vi "sub_list_all_devices_for_user_flat_output.vi"(8 "error in (no error)":errorcluster, 11 "daq.io type in":T2={"daq.io ref"=refnum, "daq.io API Base"="http://dashboard.daq.io/api/v1", "Device Type Key"="", "Device Key"="", "Account ID"="", "online"=FALSE, "SSL"=TRUE}) -> (0 "error out":errorcluster, 2 "List of Devices":T1[](array[typedef]), 3 "daq.io type out":T2={"daq.io ref"=refnum, "daq.io API Base"="http://dashboard.daq.io/api/v1", "Device Type Key"="", "Device Key"="", "Account ID"="", "online"=FALSE, "SSL"=TRUE})   [LabVIEW 2013, in "daqio minimal.lvlib"]
doc: "This VI returns a flat list of devices and their corresponding device types"
uses:
  daqio minimal.lvlib
  _typedefs/daqio-Type.ctl
  <vilib>/httpClient/ClientHandle.ctl
  _typedefs/daqio-Device-Specifier.ctl
  _typedefs/FGV_commands.ctl
  <vilib>/httpClient/LabVIEWHTTPClient.lvlib
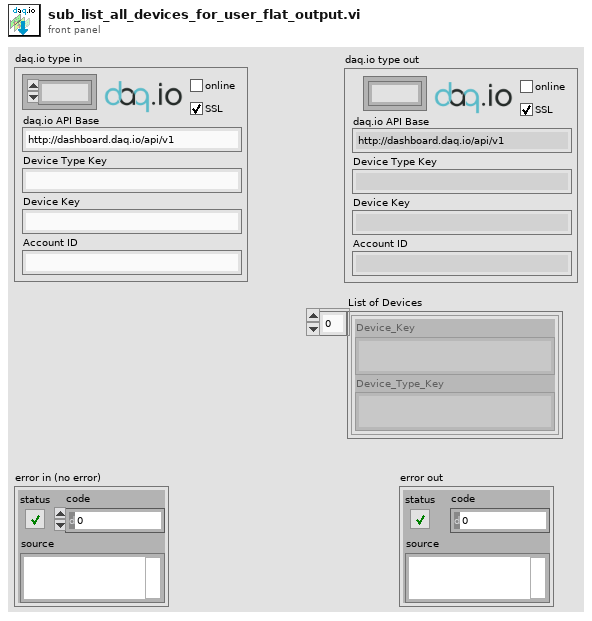
[diagram p1: front panel]
types:
  T1 = typedef "daqio minimal.lvlib/daqio-Device-Specifier.ctl" = cluster{"Device_Key":string, "Device_Type_Key":string}
  T2 = typedef "daqio minimal.lvlib/daqio-Type.ctl" = cluster{"daq.io ref":T3, "daq.io API Base":string, "Device Type Key":string, "Device Key":string, "Account ID":string, "online":bool, "SSL":bool}
  T3 = typedef "LabVIEWHTTPClient.lvlib/ClientHandle.ctl" = refnum<k1>
  T4 = typedef "daqio minimal.lvlib/FGV_commands.ctl" = enum16{"Init / Update", "Read From File", "Edit Item", "Find or Add Item", "Remove Item", "Delete All"}
  T5 = typedef "daqio minimal.lvlib/daqio-Device-Type-Info-return.ctl" = cluster{"channel_types":T6[], "devices":T7[], "label":string, "event_types":T8[], "key":string, "tag_types":T9[], "id":string, "permissions":cluster{"write":string[], "read":string[]}}
  T6 = typedef "daqio minimal.lvlib/daqio-Channel-Type-POST-return.ctl" = cluster{"device_type_id":string, "id":string, "key":string, "label":string, "data_type":string, "permissions":cluster{"write":string[], "read":string[]}}
  T7 = typedef "daqio minimal.lvlib/daqio-Device.ctl" = cluster{"permissions":cluster{"write":string[], "read":string[]}, "id":string, "label":string, "key":string, "device_type_id":string, "tags":cluster{"key":string, "value":string}[], "files":string[]}
  T8 = typedef "daqio minimal.lvlib/daqio-Event-Type.ctl" = cluster{"device_type_id":string, "permissions":cluster{"read":string[], "write":string[]}, "id":string, "key":string, "label":string}
  T9 = typedef "daqio minimal.lvlib/daqio-Tag-Type-POST-return.ctl" = cluster{"label":string, "id":string, "device_type_id":string, "permissions":cluster{"write":string[], "read":string[]}, "default":string, "key":string}
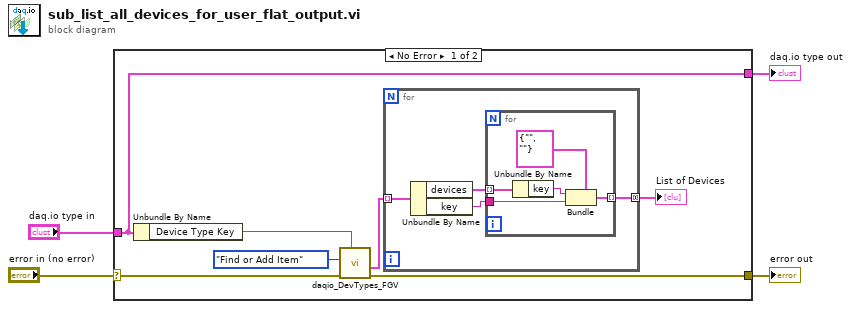
[diagram p0: block diagram]
diagram:
  n1 = case shown="No Error" "error in (no error)" {
    selector: "error in (no error)" -> [w9 w21]
    tunnel: [w10 w21] -> w3
    tunnel: "daq.io type in" -> [w7 w22]
    tunnel: [w7 w22] -> w1
    frame No Error {
      n2 = Unbundle By Name(w7) -> ("Device Type Key"=w8:string)
      n3 = call "daqio_DevTypes_FGV.vi"("Dev Type Key"=w8, "error in (no error)"=w9, "Action"=FGV_commands."Find or Add Item") -> ("error out"=w10:errorcluster, "Dev Types out"=w6:T5[])  [unwired: 4 in, 3 out]
      n4 = for {
        tunnel: w6 -> [w15] mode=indexing
        tunnel: [w13] -> w5 mode=concatenating
        n5 = Unbundle By Name(w15) -> ("devices"=w14:T7[], "key"=w12:string)
        n6 = for {
          tunnel: w14 -> [w20] mode=indexing
          tunnel: [w19] -> w13 mode=indexing
          tunnel: w12 -> [w18]
          n7 = Unbundle By Name(w20) -> ("key"=w17:string)
          n8 = Bundle(cluster=T1 {"Device_Key"="", "Device_Type_Key"=""} ("Device to switch to"), "Device_Key"=w17, "Device_Type_Key"=w18) -> (w19:T1)
        }
      }
      "List of Devices" <- w5
    }
    frame Error {
    }
  }
  "error out" <- w3
  "daq.io type out" <- w1
